vi "ValueAsInt.vi"(8 "error in (no error)":errorcluster, 11 "Parameter":string="  <value><int>123</int></value>\n    ") -> (0 "error out":errorcluster, 3 "value":i32)   [LabVIEW 2009]
doc: "Convert XML-RPC integer to LV integer (I32)"
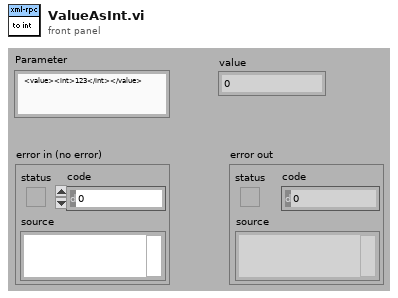
[diagram p1: front panel]
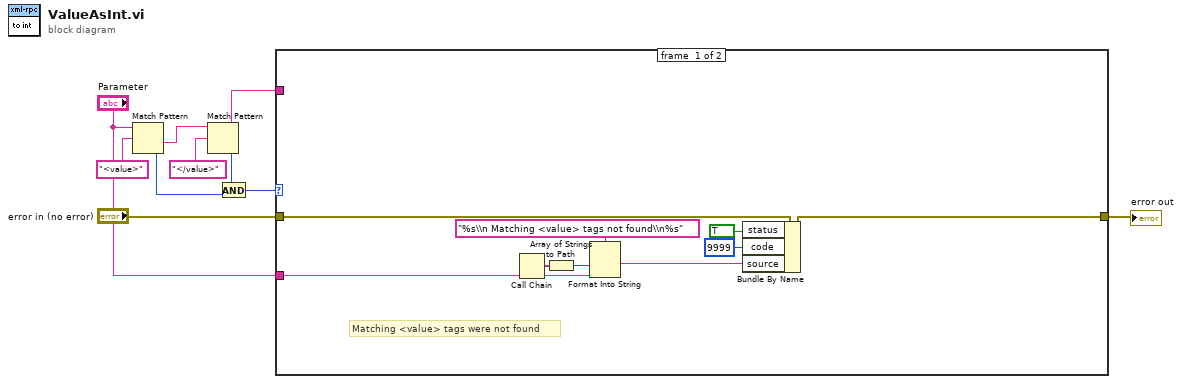
[diagram p0: block diagram]
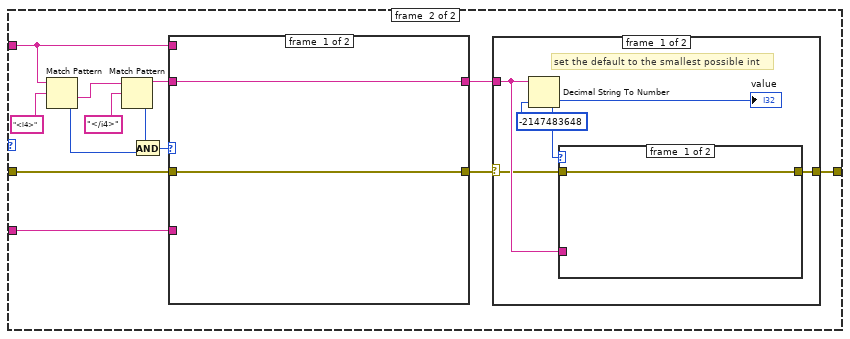
[diagram p2: hidden frame]
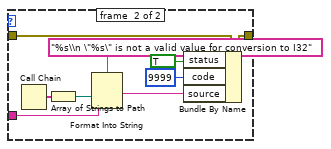
[diagram p3: hidden frame]
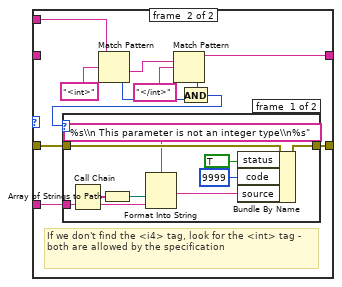
[diagram p5: hidden frame]
diagram:
  n1 = Match Pattern(string="Parameter", regular expression="<value>") -> (after substring=w9:string, offset past match=w2:i32)  [unwired: 1 in, 2 out]
  n2 = Match Pattern(string=w9, regular expression="</value>") -> (before substring=w7:string, offset past match=w3:i32)  [unwired: 1 in, 2 out]
  n3 = And(x=w3, y=w2) -> (x .and. y?=w1:i32)
  n4 = case shown="Default" w1 {
    tunnel: w7 -> [_ w29]
    tunnel: "error in (no error)" -> [w13 w27]
    tunnel: [w12 w22] -> w5
    tunnel: "Parameter" -> [w16 w26]
    frame #0 {
      # "Matching <value> tags were not found"
      n5 = Call Chain() -> (call chain=w19:string[])
      n6 = Array of Strings to Path(0:w19) -> (2:w18:path)  [unwired: 1 in]
      n7 = Format Into String(format string="%s\\n Matching <value> tags not found\\n%s", w18, w16) -> (resulting string=w11:string)  [unwired: 2 in, 1 out]
      n8 = Bundle By Name(cluster=w13, "status"=TRUE, "code"=9999, "source"=w11) -> (w12:errorcluster)
    }
    frame #1 {
      n9 = Match Pattern(string=w29, regular expression="<i4>") -> (after substring=w31:string, offset past match=w24:i32)  [unwired: 1 in, 2 out]
      n10 = Match Pattern(string=w31, regular expression="</i4>") -> (before substring=w28:string, offset past match=w25:i32)  [unwired: 1 in, 2 out]
      n11 = And(x=w25, y=w24) -> (x .and. y?=w23:i32)
      n12 = case shown="Default" w23 {
        tunnel: w29 -> [_ w58]
        tunnel: w28 -> [w50 _]
        tunnel: [w50 w51] -> w21
        tunnel: w27 -> [w49 w57]
        tunnel: [w49 w56] -> w20
        tunnel: w26 -> [_ w55]
        frame #0 {
        }
        frame #1 {
          # "If we don't find the <i4> tag, look for the <int> tag - both are allowed by the specification"
          n13 = Match Pattern(string=w58, regular expression="<int>") -> (after substring=w60:string, offset past match=w52:i32)  [unwired: 1 in, 2 out]
          n14 = Match Pattern(string=w60, regular expression="</int>") -> (before substring=w51:string, offset past match=w53:i32)  [unwired: 1 in, 2 out]
          n15 = And(x=w53, y=w52) -> (x .and. y?=w54:i32)
          n16 = case shown="-1" w54 {
            tunnel: w57 -> [w69 w71]
            tunnel: [w68 w71] -> w56
            tunnel: w55 -> [w63 _]
            frame #0 {
              n17 = Call Chain() -> (call chain=w70:string[])
              n18 = Array of Strings to Path(0:w70) -> (2:w65:path)  [unwired: 1 in]
              n19 = Format Into String(format string="%s\\n This parameter is not an integer type\\n%s", w65, w63) -> (resulting string=w64:string)  [unwired: 2 in, 1 out]
              n20 = Bundle By Name(cluster=w69, "status"=TRUE, "code"=9999, "source"=w64) -> (w68:errorcluster)
            }
            frame #1 {
            }
          }
        }
      }
      n21 = case shown="Error" w20 {
        selector: w20 -> [w33 w48]
        tunnel: [w36 w48] -> w22
        tunnel: w21 -> [w35 _]
        frame #0 {
          # "set the default to the smallest possible int"
          n22 = Decimal String To Number(string=w35, default (0L)=-2147483648 ("Numeric")) -> (number=w34:i32)  [unwired: 1 in, 1 out]
          "value" <- w34
          n23 = case shown="-2147483648" w34 {
            tunnel: w33 -> [w38 w42]
            tunnel: [w38 w41] -> w36
            tunnel: w35 -> [_ w40]
            frame #0 {
            }
            frame #1 {
              n24 = Call Chain() -> (call chain=w43:string[])
              n25 = Array of Strings to Path(0:w43) -> (2:w46:path)  [unwired: 1 in]
              n26 = Format Into String(format string="%s\\n \"%s\" is not a valid value for conversion to I32", w46, w40) -> (resulting string=w47:string)  [unwired: 2 in, 1 out]
              n27 = Bundle By Name(cluster=w42, "status"=TRUE, "code"=9999, "source"=w47) -> (w41:errorcluster)
            }
          }
        }
        frame #1 {
          # "don't try to convert if we don't find a valid tag"
        }
      }
    }
  }
  "error out" <- w5
